vi "DataManipulation.vi"(9 "y3":i32, 10 "y 2":i32, 11 "y":i32) -> (3 "Data out":u32)   [LabVIEW 2022 SP3, in "BME680.lvlib" / "BME680.lvclass"]
uses:
  BME680.lvclass
  BME680.lvclass/BME680.ctl
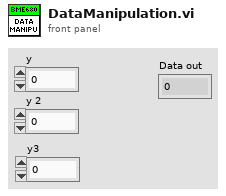
[diagram p1: front panel]
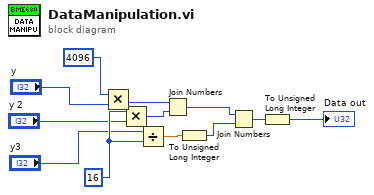
[diagram p0: block diagram]
diagram:
  w9 = 16
  n1 = Multiply(x=4096, y="y") -> (x*y=w11:i32)
  n2 = Multiply(x=w9, y="y 2") -> (x*y=w10:i32)
  n3 = Divide(x="y3", y=w9) -> (x/y=w7:dbl)
  n4 = Join Numbers(hi=w11, lo=w10) -> ((hi.lo)=w8:u64)
  n5 = To Unsigned Long Integer(number=w7) -> (unsigned 32bit integer=w6:u32)
  n6 = Join Numbers(hi=w8, lo=w6) -> ((hi.lo)=w2:u64)
  n7 = To Unsigned Long Integer(number=w2) -> (unsigned 32bit integer=→"Data out":u32)
